vi "Error_Control.vi"(0 "GEA2":T3, 1 "ERD Loop":T4, 2 "Command (Handle Errors)":T2=enum."Handle Errors", 5 "Receive Loop Error":T7, 7 "UI Loop Error":T6, 9 "DAQ":T5, 11 "Error In":errorcluster, 12 "Cont Send":T1) -> (15 "Error Out":errorcluster)   [LabVIEW 2014]
uses:
  type defs/Ref_ReceiveLoop_UserEvent.ctl
  type defs/Ref_UILoop_UserEvent.ctl
  type defs/Ref_DAQ_Queue.ctl
  type defs/DAQ_States.ctl
  type defs/Ref_ERD_Queue.ctl
  type defs/ERD_Data_Loop_Control.ctl
  type defs/Ref_GEA2_Queue.ctl
  Utility/Labview GEA2 Toolkit v2.1/GExplorer Support/typedefs/GExplorer_Data_Cluster.ctl
  type defs/Error_Command.ctl
  type defs/Ref_Cont_Send_Queue.ctl
  type defs/Cont_Send_States.ctl
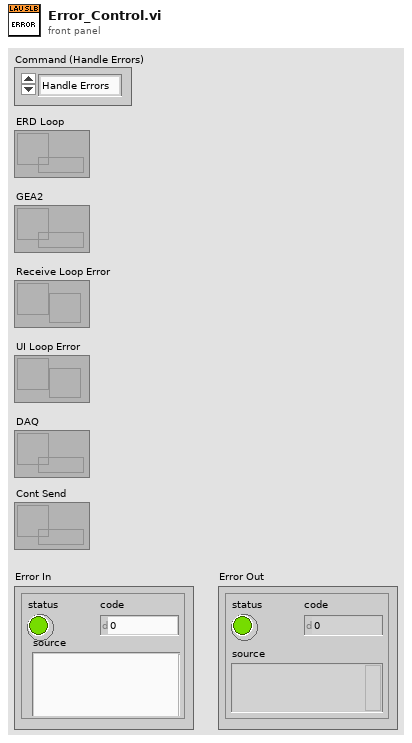
[diagram p1: front panel]
types:
  T1 = typedef "Ref_Cont_Send_Queue.ctl" = refnum<queue>
  T2 = typedef "Error_Command.ctl" = enum16{"Initialize", "Handle Errors", "Report Errors"}
  T3 = typedef "Ref_GEA2_Queue.ctl" = refnum<queue>
  T4 = typedef "Ref_ERD_Queue.ctl" = refnum<queue>
  T5 = typedef "Ref_DAQ_Queue.ctl" = refnum<queue>
  T6 = typedef "Ref_UILoop_UserEvent.ctl" = refnum<user-event>
  T7 = typedef "Ref_ReceiveLoop_UserEvent.ctl" = refnum<user-event>
  T8 = typedef "Cont_Send_States.ctl" = enum16{"Run", "Shutdown"}
  T9 = typedef "DAQ_States.ctl" = enum16{"Wait for Init", "Verify Hardware", "Initialize", "Run", "Shutdown", "Exit"}
  T10 = typedef "ERD_Data_Loop_Control.ctl" = cluster{"Data":variant, "State":enum16{"Run", "Shutdown"}}
  T11 = typedef "GExplorer_Data_Cluster.ctl" = cluster{"Data":variant, "State":enum16{"Add to Log", "Clear", "Shutdown"}}
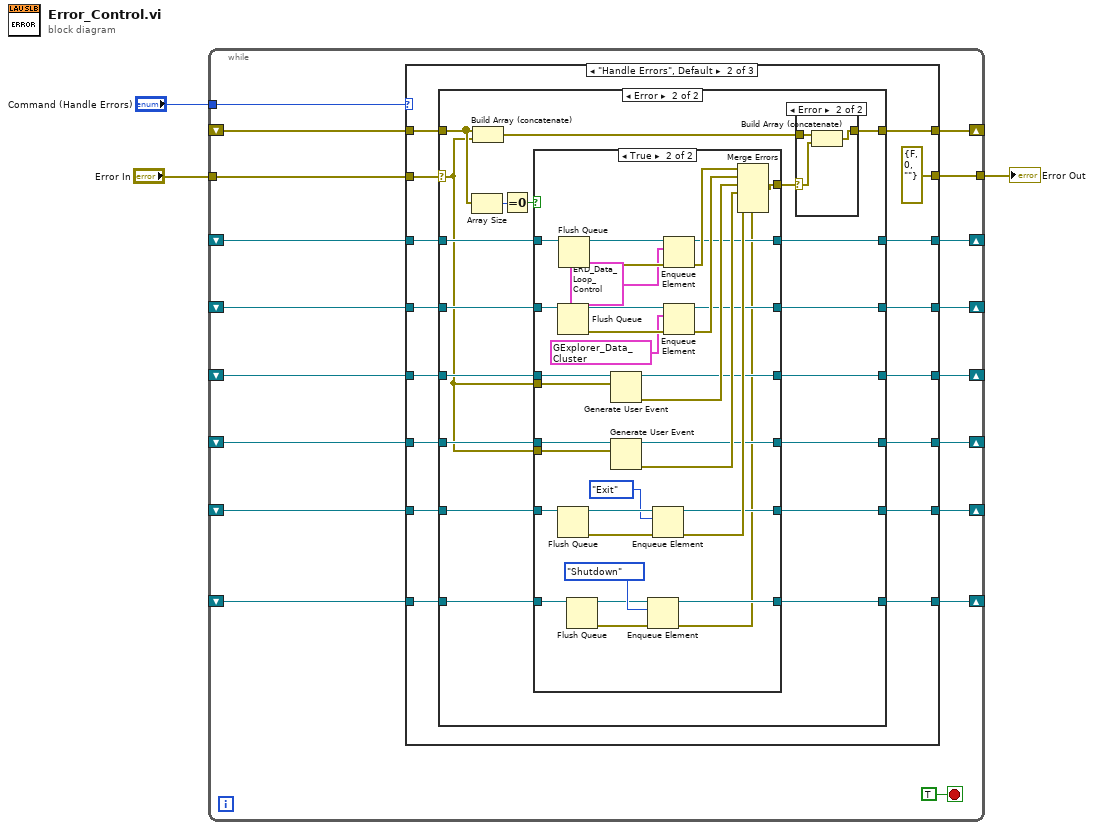
[diagram p0: block diagram]
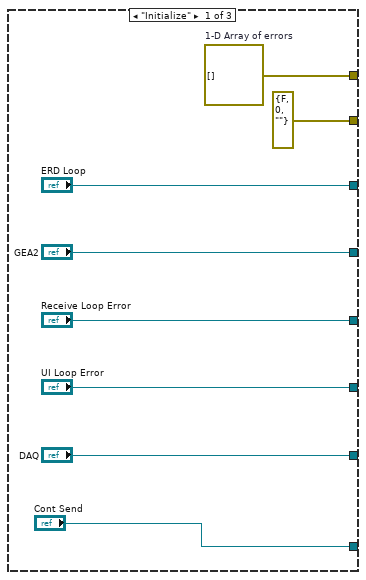
[diagram p2: hidden frame]
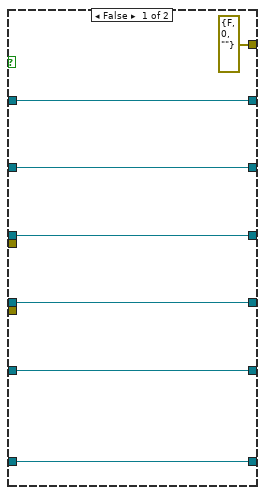
[diagram p4: hidden frame]
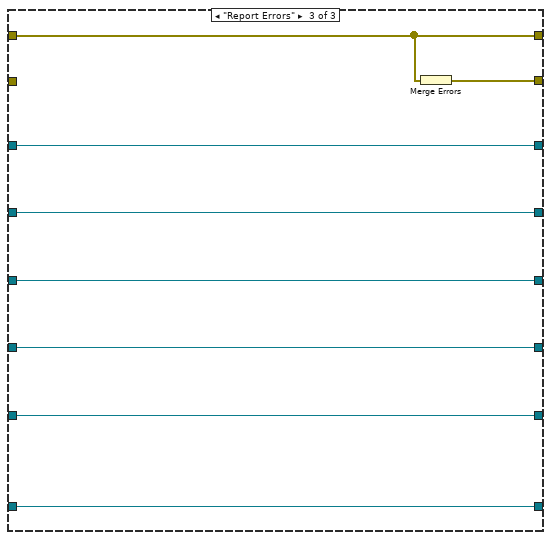
[diagram p6: hidden frame]
diagram:
  n1 = while {
    tunnel: "Error In" -> [w19]
    tunnel: "Command (Handle Errors)" -> [w20]
    shift-right: [w18] -> _
    shift-left: _ -> [w17]
    tunnel: [w16] -> w1
    shift-right: [w15] -> _
    shift-left: _ -> [w10]
    shift-right: [w14] -> _
    shift-left: _ -> [w9]
    shift-right: [w13] -> _
    shift-left: _ -> [w8]
    shift-right: [w12] -> _
    shift-left: _ -> [w7]
    shift-right: [w11] -> _
    shift-left: _ -> [w6]
    shift-right: [w5] -> _
    shift-left: _ -> [w4]
    stop <- TRUE stop-if-true
    n2 = case shown="\"Handle Errors\", Default" w20 {
      tunnel: w19 -> [_ w45 _]
      tunnel: [w29 w38 w122] -> w18
      tunnel: w17 -> [_ w44 w122]
      tunnel: [errorcluster {"status"=FALSE, "code"=0, "source"=""} ("Error In") errorcluster {"status"=FALSE, "code"=0, "source"=""} ("Error In") w123] -> w16
      tunnel: ["ERD Loop" w36 w121] -> w15
      tunnel: ["GEA2" w37 w120] -> w14
      tunnel: ["Receive Loop Error" w35 w119] -> w13
      tunnel: ["UI Loop Error" w34 w118] -> w12
      tunnel: ["DAQ" w33 w117] -> w11
      tunnel: w10 -> [_ w43 w121]
      tunnel: w9 -> [_ w42 w120]
      tunnel: w8 -> [_ w41 w119]
      tunnel: w7 -> [_ w40 w118]
      tunnel: w6 -> [_ w39 w117]
      tunnel: ["Cont Send" w30 w116] -> w5
      tunnel: w4 -> [_ w31 w116]
      frame "Initialize" {
        w29 = errorcluster[] []  # 1-D Array of errors
      }
      frame "Handle Errors", Default {
        n3 = case shown="Error" w45 {
          selector: w45 -> [_ w61]
          tunnel: w44 -> [w52 w71]
          tunnel: w43 -> [w51 w68]
          tunnel: w42 -> [w50 w67]
          tunnel: w41 -> [w49 w66]
          tunnel: w40 -> [w48 w65]
          tunnel: w39 -> [w47 w64]
          tunnel: [w52 w62] -> w38
          tunnel: [w50 w60] -> w37
          tunnel: [w51 w59] -> w36
          tunnel: [w49 w58] -> w35
          tunnel: [w48 w57] -> w34
          tunnel: [w47 w56] -> w33
          tunnel: w31 -> [w46 w54]
          tunnel: [w46 w53] -> w30
          frame No Error {
          }
          frame Error {
            n4 = Array Size(array=w71) -> (size(s)=w70:i32)
            n5 = Build Array (concatenate)(w71, w61) -> (w55:errorcluster[])
            n6 = Equal To 0?(x=w70) -> (x = 0?=w69:bool)
            n7 = case shown="True" w69 {
              tunnel: w68 -> [w77 w111]
              tunnel: w67 -> [w76 w110]
              tunnel: w66 -> [w75 w101]
              tunnel: w65 -> [w74 w99]
              tunnel: w64 -> [w73 w109]
              tunnel: [errorcluster {"status"=FALSE, "code"=0, "source"=""} ("error IO") w108] -> w63
              tunnel: w61 -> [_ w100]
              tunnel: w61 -> [_ w98]
              tunnel: [w76 w89] -> w60
              tunnel: [w77 w88] -> w59
              tunnel: [w75 w87] -> w58
              tunnel: [w74 w86] -> w57
              tunnel: [w73 w85] -> w56
              tunnel: w54 -> [w72 w83]
              tunnel: [w72 w81] -> w53
              frame False {
              }
              frame True {
                n8 = Flush Queue(queue=w110) -> (queue out=w106:T3, error out=w107:errorcluster)  [unwired: 1 in, 1 out]
                n9 = Flush Queue(queue=w109) -> (queue out=w97:T5, error out=w95:errorcluster)  [unwired: 1 in, 1 out]
                n10 = Flush Queue(queue=w111) -> (queue out=w103:T4, error out=w104:errorcluster)  [unwired: 1 in, 1 out]
                n11 = Flush Queue(queue=w83) -> (queue out=w82:T1, error out=w80:errorcluster)  [unwired: 1 in, 1 out]
                n12 = Generate User Event(user event=w101, event data cluster=w100) -> (user event out=w87:T7, error out=w92:errorcluster)  [unwired: 2 in]
                n13 = Generate User Event(user event=w99, event data cluster=w98) -> (user event out=w86:T6, error out=w93:errorcluster)  [unwired: 2 in]
                n14 = Enqueue Element(queue=w82, element=Cont_Send_States."Shutdown", error in (no error)=w80) -> (queue out=w81:T1, error out=w79:errorcluster)  [unwired: 1 in, 1 out]
                n15 = Enqueue Element(queue=w97, element=DAQ_States."Exit", error in (no error)=w95) -> (queue out=w85:T5, error out=w94:errorcluster)  [unwired: 1 in, 1 out]
                n16 = Enqueue Element(queue=w103, element=T10 {"Data"=variant, "State"=enum."Shutdown"}, error in (no error)=w104) -> (queue out=w88:T4, error out=w91:errorcluster)  [unwired: 1 in, 1 out]
                n17 = Enqueue Element(queue=w106, element=T11 {"Data"=variant, "State"=enum."Shutdown"}, error in (no error)=w107) -> (queue out=w89:T3, error out=w90:errorcluster)  [unwired: 1 in, 1 out]
                n18 = Merge Errors(w91, w90, w92, w93, w94, w79) -> (w108:errorcluster)
              }
            }
            n19 = case shown="Error" w63 {
              selector: w63 -> [_ w114]
              tunnel: [w112 w115] -> w62
              tunnel: w55 -> [w112 w113]
              frame No Error {
              }
              frame Error {
                n20 = Build Array (concatenate)(w113, w114) -> (w115:errorcluster[])
              }
            }
          }
        }
      }
      frame "Report Errors" {
        n21 = Merge Errors(w122) -> (w123:errorcluster)
      }
    }
  }
  "Error Out" <- w1
